vi "find device.vi"(8 "error in (no error)":errorcluster, 11 "all device":T1) -> (0 "error out":errorcluster, 3 "all device out":T1)   [LabVIEW 2011]
uses:
  C:/Program Files/National Instruments/LabVIEW 8.6/resource/objmgr/daqmx.rc
  chanel.ctl
  signal type.ctl
  gain.ctl
  single chanel.ctl
  CARD config.ctl
  filter.ctl
  Power_config.ctl
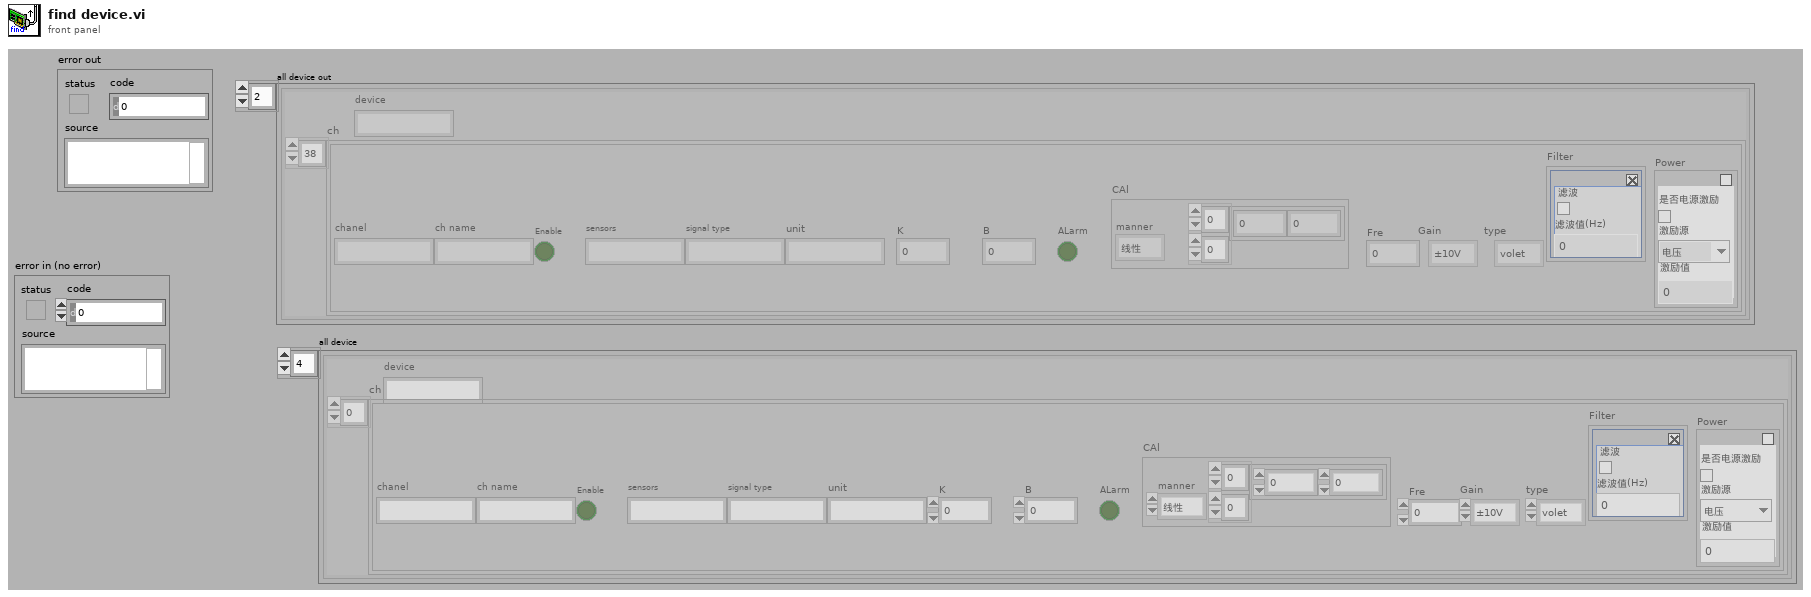
[diagram p1: front panel]
types:
  T1 = typedef "chanel.ctl" = T2[]
  T2 = typedef "CARD config.ctl" = cluster{"device":string, "ch":T3[]}
  T3 = typedef "single chanel.ctl" = cluster{"chanel":string, "ch name":string, "Enable":bool, "sensors":string, "signal type":string, "unit":string, "K":dbl, "B":dbl, "ALarm":bool, "CAl":cluster{"manner":enum16{"线性", "查表"}, "data":dbl[][]}, "Fre":dbl, "type":T4, "Gain":T5, "Filter":T6, "Power":T7}
  T4 = typedef "signal type.ctl" = enum16{"未设置", "volet", "current", "vibration", "electric charge ", "resistance "}
  T5 = typedef "gain.ctl" = enum16{"±10V", "±5V", "±2.5V", "±1V", "±500mV", "±100mV", "10V", "5V", "2.5V", "1V", "500mV", "100mV"}
  T6 = typedef "filter.ctl" = cluster{"en":bool, "value":i32, "Boolean":bool}
  T7 = typedef "Power_config.ctl" = cluster{"power_en":bool, "Mode":enum16{"电压", "电流"}, "value":dbl, "Boolean":bool}
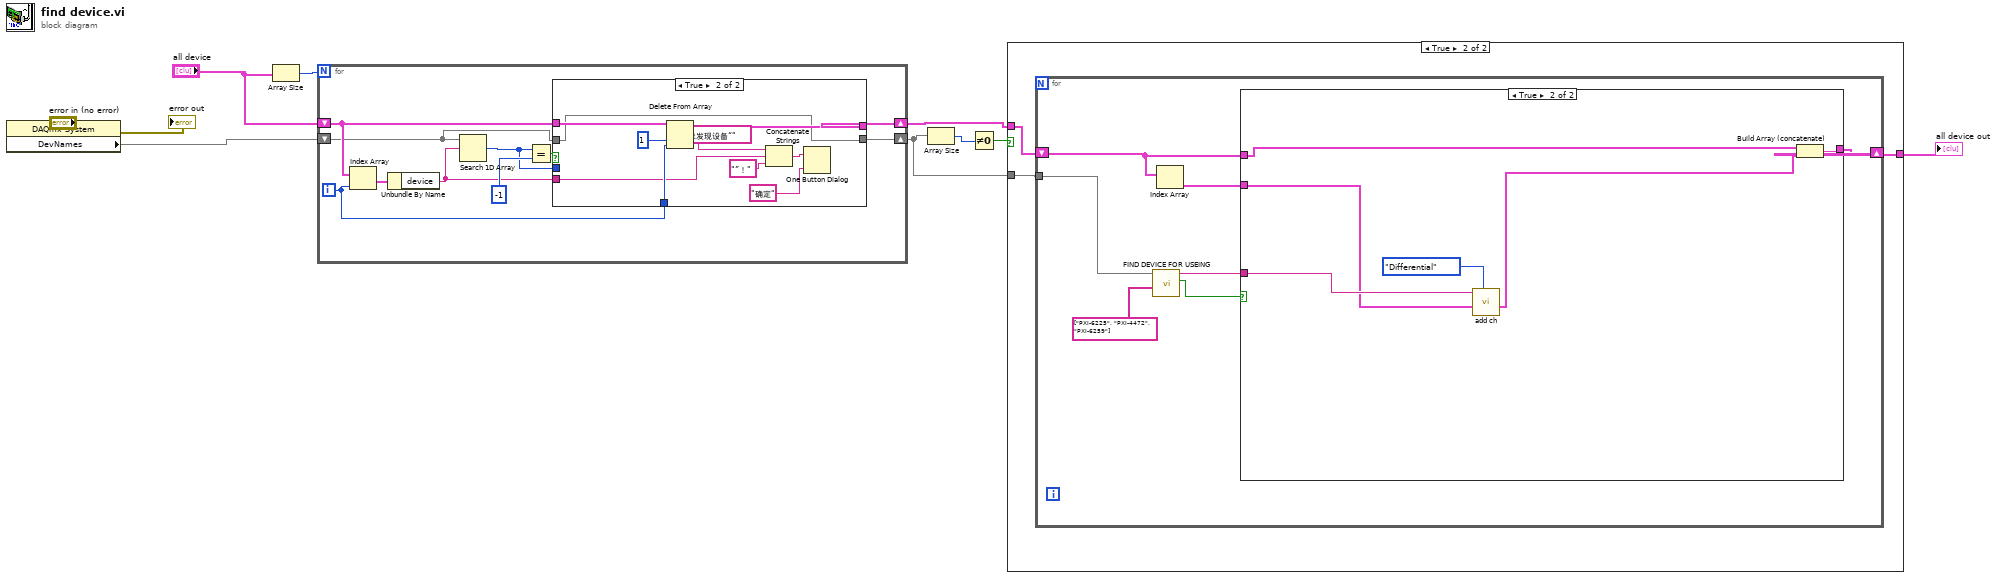
[diagram p0: block diagram]
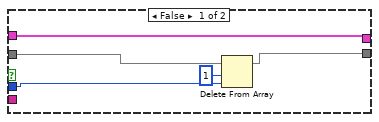
[diagram p4: hidden frame]
diagram:
  n1 = property class="DAQmx System"(error in="error in (no error)") -> (error out=→"error out":errorcluster, "DevNames"=w10)  [unwired: 1 in, 1 out]
  n2 = Array Size(array="all device") -> (size(s)=w9:i32)
  n3 = for {
    N: w9 -> [_]
    shift-right: [w15] -> w3
    shift-left: "all device" -> [w17]
    shift-right: [w11] -> w2
    shift-left: w10 -> [w13]
    i -> [w16]
    n4 = Index Array(array=w17, index=w16) -> (element=w19:T2)
    n5 = Unbundle By Name(w19) -> ("device"=w14:string)
    n6 = Search 1D Array(1D array=w13, element=w14) -> (index of element=w12:i32)  [unwired: 1 out]
    n7 = Equal?(x=w12, y=-1) -> (x = y?=w18:bool)
    n8 = case shown="True" w18 {
      tunnel: w17 -> [w25 w35]
      tunnel: w16 -> [_ w33]
      tunnel: [w25 w32] -> w15
      tunnel: w14 -> [_ w28]
      tunnel: w13 -> [w24 w26]
      tunnel: w12 -> [w23 _]
      tunnel: [w21 w26] -> w11
      frame False {
        n9 = Delete From Array(array=w24, length=1, index=w23) -> (array with subset deleted=w21)  [unwired: 1 out]
      }
      frame True {
        n10 = Delete From Array(array=w35, length=1, index=w33) -> (array with subset deleted=w32:T1)  [unwired: 1 out]
        n11 = Concatenate Strings("未发现设备“" ("string"), w28, "”！" ("string")) -> (w30:string)
        n12 = One Button Dialog(message=w30, button name ("OK")="确定") -> ()  [unwired: 1 out]
      }
    }
  }
  n13 = Array Size(array=w2) -> (size(s)=w5:i32)
  n14 = Not Equal To 0?(x=w5) -> (x != 0?=w4:bool)
  n15 = case shown="True" w4 {
    tunnel: w3 -> [w36 w38]
    tunnel: w2 -> [_ w39]
    tunnel: [w36 w37] -> w1
    frame False {
    }
    frame True {
      n16 = for {
        tunnel: w39 -> [w46]
        shift-right: [w41] -> w37
        shift-left: w38 -> [w43]
        n17 = call "FIND DEVICE FOR USEING.vi"("product type"=string[] ["PXI-6225", "PXI-4472", "PXI-6259"], "DAQmx Device Name"=w46) -> ("T button?"=w40:bool, "DAQmx Device Name OUT"=w44:tag)  [unwired: 8 out]
        n18 = Index Array(array=w43) -> (element=w42:T2)  [unwired: 1 in]
        n19 = case shown="True" w40 {
          tunnel: [w47 w53] -> w41
          tunnel: w44 -> [_ w52]
          tunnel: w43 -> [w47 w50]
          tunnel: w42 -> [_ w49]
          frame False {
          }
          frame True {
            n20 = call "add ch.vi"("tem"=enum16{"Single-Ended", "Differential"}."Differential", "output cluster"=w49, "DAQmx Device Name OUT"=w52) -> ("input cluster"=w48:T2)  [unwired: 8 out]
            n21 = Build Array (concatenate)(w50, w48) -> (w53:T1)
          }
        }
      }
    }
  }
  "all device out" <- w1
